vi "PI_Loop.vi"(8 "ki":dbl=0.01, 9 "kp":dbl=0.2, 10 "integral":dbl, 11 "diff":dbl) -> (3 "update":dbl)   [LabVIEW 2019]
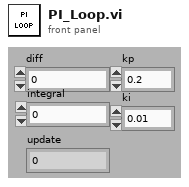
[diagram p1: front panel]
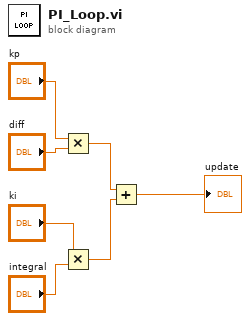
[diagram p0: block diagram]
diagram:
  n1 = Multiply(x="kp", y="diff") -> (x*y=w5:dbl)
  n2 = Multiply(x="ki", y="integral") -> (x*y=w4:dbl)
  n3 = Add(x=w5, y=w4) -> (x+y=→"update":dbl)
